vi "Memory.Array.Create.vi"(8 "error in (no error)":errorcluster) -> (0 "error out":errorcluster, 3 "Array out":refnum<class "Memory.Array.lvclass">)   [LabVIEW 2016, in "LabVIEW Memory Manager.lvlib" / "Memory.Array.lvclass"]
uses:
  Memory.Array.lvclass
  Memory.Array.lvclass/Memory.Array.ctl
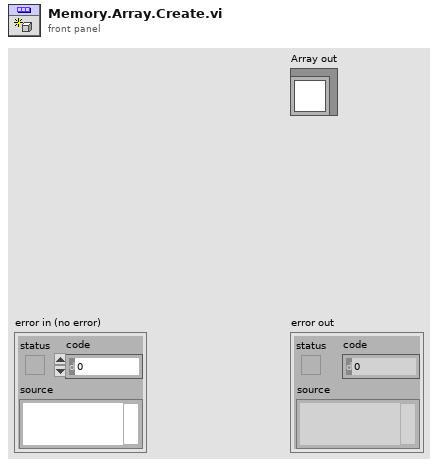
[diagram p1: front panel]
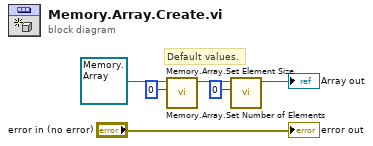
[diagram p0: block diagram]
diagram:
  # "Default values."
  n1 = call "Memory.Array.Set Element Size.vi"("size of element"=i64 0, "Memory.Array in"=refnum<class "Memory.Array.lvclass"> refnum ("LabVIEW Memory Manager.lvlib:Array")) -> ("Memory.Array out"=w6:refnum<class "Memory.Array.lvclass">)  [unwired: 8 in, 1 out]
  n2 = call "Memory.Array.Set Number of Elements.vi"("number of elements"=u64 0, "Memory.Array in"=w6) -> ("Memory.Array out"=→"Array out":refnum<class "Memory.Array.lvclass">)  [unwired: 8 in, 1 out]
  "error out" <- "error in (no error)"
